vi "DuplicateHandler.vi"(6 "Abort?":bool, 8 "error in":errorcluster, 10 "NewFileName":path, 11 "current file":string) -> (0 "error out":errorcluster, 4 "Abort out":bool)   [LabVIEW 2023]
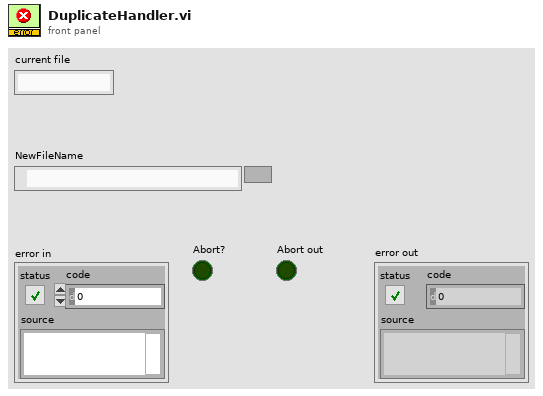
[diagram p1: front panel]
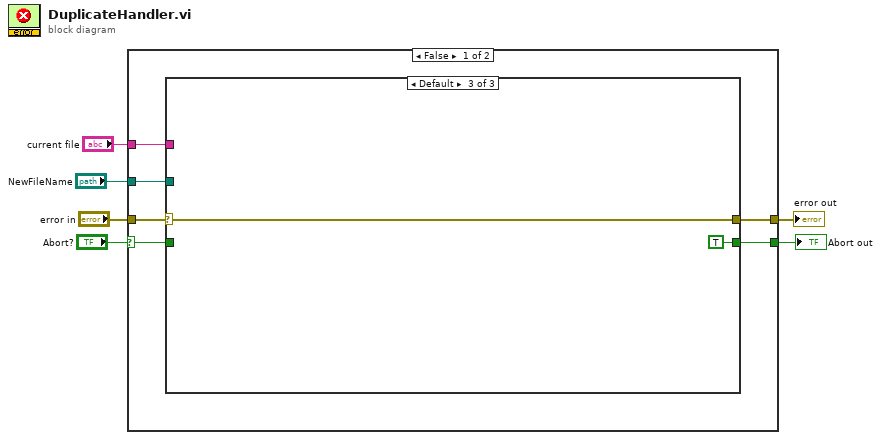
[diagram p0: block diagram]
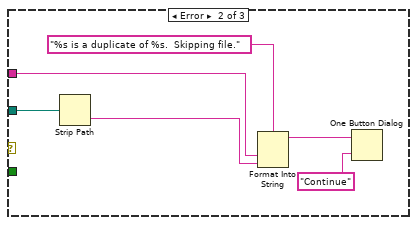
[diagram p3: hidden frame]
diagram:
  n1 = case shown="False" "Abort?" {
    selector: "Abort?" -> [w9 w24]
    tunnel: "error in" -> [w12 w23]
    tunnel: [w10 w24] -> w4
    tunnel: [w11 w23] -> w3
    tunnel: "NewFileName" -> [w8 _]
    tunnel: "current file" -> [w7 _]
    frame False {
      n2 = case shown="Default" w12 {
        selector: w12 -> [w14 _ w22]
        tunnel: [w14 _ w22] -> w11
        tunnel: [w13 _ TRUE] -> w10
        tunnel: w9 -> [w13 _ _]
        tunnel: w8 -> [_ w20 _]
        tunnel: w7 -> [_ w18 _]
        frame No Error {
        }
        frame Error {
          n3 = Strip Path(path=w20) -> (name=w17:string)  [unwired: 1 out]
          n4 = Format Into String(format string="%s is a duplicate of %s.  Skipping file.", w18, w17) -> (resulting string=w16:string)  [unwired: 2 in, 1 out]
          n5 = One Button Dialog(message=w16, button name ("OK")="Continue") -> ()  [unwired: 1 out]
        }
        frame Default {
        }
      }
    }
    frame True {
    }
  }
  "error out" <- w3
  "Abort out" <- w4
